vi "Test Missing Classes.vi"(8 "error in":errorcluster, 11 "My Computer":refnum<vi>) -> (0 "error out":errorcluster, 4 "Missing items from LabVIEW project":path[](array[path]), 5 "Pass":bool, 6 "Debug":path[](array[path]))   [LabVIEW 2020, in "Missing in Project Tests.lvlib"]
doc: "Tests to make sure all classes defined in the project are saved to disk."
uses:
  Missing in Project Tests.lvlib
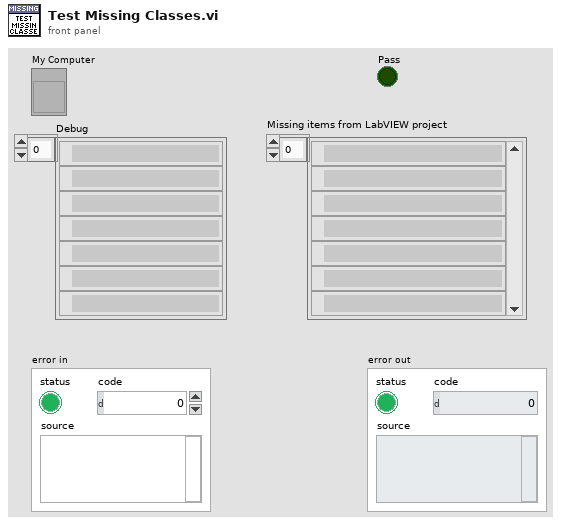
[diagram p1: front panel]
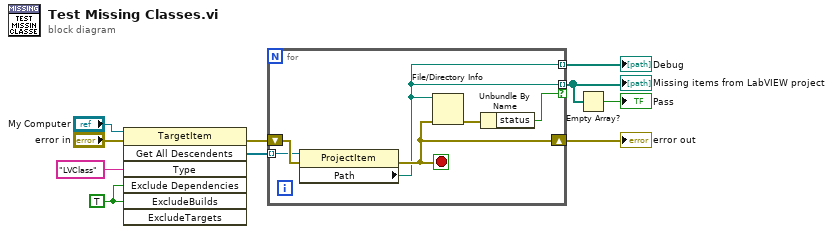
[diagram p0: block diagram]
diagram:
  w3 = TRUE ("ExcludeBuilds")
  n1 = invoke class="TargetItem" method="Get All Descendents"(reference="My Computer", error in="error in", "Type"="LVClass", "Exclude Dependencies"=w3, "ExcludeBuilds"=w3) -> (error out=w10:errorcluster, "All Descendents"=w4:refnum<vi>[])  [unwired: 2 in, 5 out]
  n2 = for {
    tunnel: w4 -> [w13] mode=indexing
    shift-right: [w14] -> w8
    shift-left: w10 -> [w15]
    tunnel: [w11] -> w5 mode=indexing if=w12
    tunnel: [w11] -> w1 mode=indexing
    stop <- w14 stop-if-true
    n3 = property class="ProjectItem"(reference=w13, error in=w15) -> (error out=w14:errorcluster, "Path"=w11:path)  [unwired: 1 out]
    n4 = File/Directory Info(path=w11, error in=w14) -> (error out=w16:errorcluster)  [unwired: 6 out]
    n5 = Unbundle By Name(w16) -> ("status"=w12:bool)
  }
  "Missing items from LabVIEW project" <- w5
  "error out" <- w8
  "Debug" <- w1
  n6 = Empty Array?(array=w5) -> (empty?=→"Pass":bool)
